vi "Wheel__Speed.vi"() -> ()   [LabVIEW 2017]
panel:
  out "error out":errorcluster
  in  "error in":errorcluster
  out "Velocity(mph)":dbl
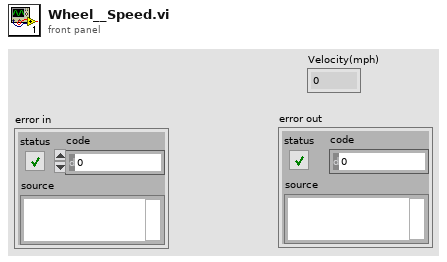
[diagram p1: front panel]
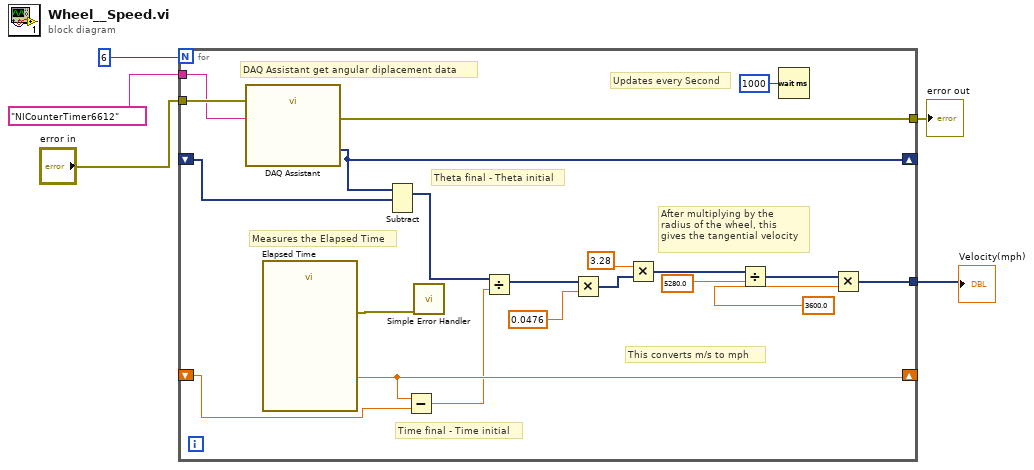
[diagram p0: block diagram]
diagram:
  n1 = for {
    N: 6 -> [_]
    shift-right: [w24] -> _
    shift-left: _ -> [w25]
    shift-right: [w23] -> _
    shift-left: _ -> [w22]
    tunnel: [w9] -> w2
    tunnel: [w8] -> w5
    tunnel: "error in" -> [w7]
    tunnel: tag "NICounterTimer6612" ("device name") -> [w6]
    # "Updates every Second"
    # "After multiplying by the\nradius of the wheel, this\ngives the tangential velocity"
    # "This converts m/s to mph"
    # "Time final - Time initial"
    # "Measures the Elapsed Time"
    # "Theta final - Theta initial"
    # "DAQ Assistant get angular diplacement data"
    n2 = call "DAQ Assistant"("error in"=w7, "device name"=w6) -> ("data"=w24:dynamicdata, "error out"=w9:errorcluster)  [unwired: 14 in, 2 out]
    n3 = call "Elapsed Time"() -> ("Elapsed Time (s)"=w23:dbl, "error out"=w10:errorcluster)  [unwired: 12 in, 6 out]
    n4 = Subtract(1:w25, 2:w24) -> (0:w21:dynamicdata)  [unwired: 1 in, 1 out]
    n5 = Subtract(x=w23, y=w22) -> (x-y=w20:dbl)
    n6 = call <vilib>:"Simple Error Handler.vi"("error in (no error)"=w10) -> ()  [unwired: 4 in, 5 out]
    n7 = Divide(x=w21, y=w20) -> (x/y=w19:dynamicdata)
    n8 = Multiply(x=w19, y=0.0476) -> (x*y=w16:dynamicdata)
    n9 = Multiply(x=3.28, y=w16) -> (x*y=w15:dynamicdata)
    n10 = Divide(x=w15, y=5280.0) -> (x/y=w12:dynamicdata)
    n11 = Wait (ms)(milliseconds to wait=u32 1000) -> ()  [unwired: 1 out]
    n12 = Multiply(x=w12, y=3600.0) -> (x*y=w8:dynamicdata)
  }
  "Velocity(mph)" <- w5
  "error out" <- w2
